vi "generate-lv-class-items.vi"() -> ()   [LabVIEW 2023]
uses:
  <resource>/Framework/Providers/_ClassSupport/Item Initialization.ctl
  <resource>/Framework/Providers/AddClass/Add Class.lvlib
  <resource>/Framework/Providers/_ClassSupport/Class Provider Support.lvlib
panel:
  in  "LV library path":path=path "C:/tmp/uhd-classes/uhd.lvlib"
  out "error out":errorcluster
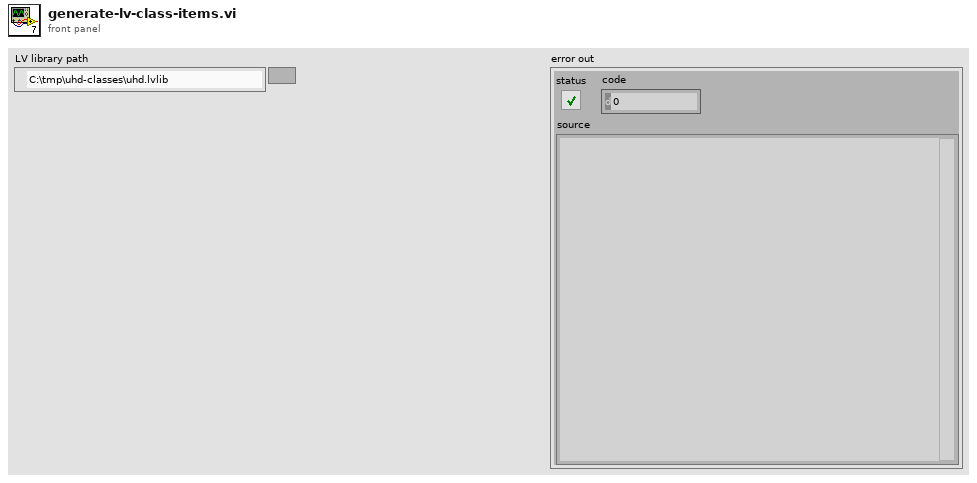
[diagram p1: front panel]
types:
  T1 = typedef "Class Provider Support.lvlib/Item Initialization.ctl" = cluster{"name":string, "folder to save":path}
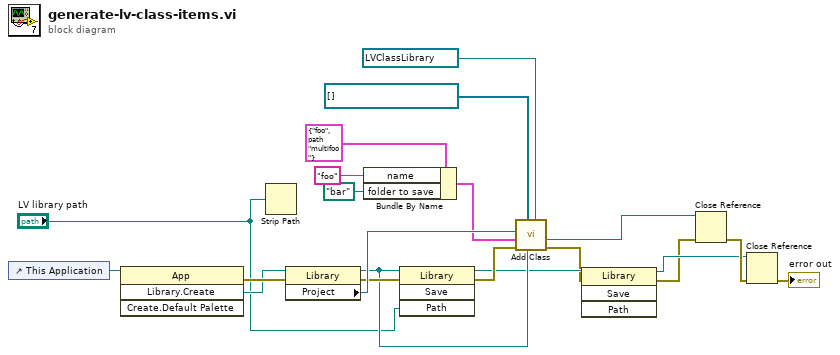
[diagram p0: block diagram]
diagram:
  n1 = control-ref of="This Application"() -> (w20:refnum<vi>)
  n2 = invoke class="App" method="Library.Create"(reference=w20) -> (error out=w19:errorcluster, "Create Library"=w18:refnum<vi>)  [unwired: 3 in, 2 out]
  n3 = Strip Path(path="LV library path") -> ()  [unwired: 2 out]
  n4 = property class="Library"(reference=w18, error in=w19) -> (reference out=w10:refnum<vi>, error out=w12:errorcluster, "Project"=w17:refnum<vi>)
  n5 = Bundle By Name(cluster=T1 {"name"="foo", "folder to save"=path "multifoo"} ("item info"), "name"="foo", "folder to save"=path "bar") -> (w6:T1)
  n6 = invoke class="Library" method="Save"(reference=w10, error in=w12, "Path"="LV library path") -> (reference out=w5:refnum<vi>, error out=w11:errorcluster)  [unwired: 1 in, 2 out]
  n7 = call <resource>:"Add Class.vi"("Class to Inherit From"=refnum<vi> refnum, "Class Owner"=w10, "Interfaces to Inherit From"=refnum<vi>[] [], "error in"=w11, "item info"=w6, "Project in"=w17) -> ("error out"=w3:errorcluster, "Created Class"=w16:refnum<vi>)  [unwired: 3 in, 1 out]
  n8 = invoke class="Library" method="Save"(reference=w5, error in=w3) -> (reference out=w4:refnum<vi>, error out=w2:errorcluster)  [unwired: 2 in, 2 out]
  n9 = Close Reference(reference=w16, error in (no error)=w2) -> (error out=w13:errorcluster)
  n10 = Close Reference(reference=w4, error in (no error)=w13) -> (error out=→"error out":errorcluster)
